vi "generate error.vi"() -> ()   [LabVIEW 2021, in "CIFCorePlugin.lvclass"]
uses:
  CIFCore/CIFCorePlugin/CIFCorePlugin.lvclass
  <vilib>/Utility/error.llb/DialogType.ctl
panel:
  out "call chain":string[](array[string])
  out "Callers' Names":string[](array[string])
  out "error out 2":errorcluster
  out "Name":string
  out "VI Name":string
  out "code out":i32 format="%0.0f"
  out "source out":string
  out "message":string=" INSTRUCTIONS:\r\rNormal Use:  When using subVIs that incorporate the error in/error out (or error I/O) structure, place this handler where you want to inform the user of an error, typically at the end of the I/O data path, as the last action of the program.  If the error in error? is ERROR, the handler creates a message describing the error and its source.  If the type of dialog = 1 (default), the message is displayed to the user, who can only acknowedge it.  If the type = 2, the user can acknowledge the message or abort execution; aborting a program with active I/O is not recommended.  If the type = 0, no message is displayed; this is used to process the error programmatically, and the error out cluster elements are wired to individual terminals for that reason.  \r\rOther Use:\n\r\nlocal testing.  To test the error code of a subVI or function that does not have the error I/O structure, you can wire its error code and a source string to the local error code and error source inputs.  If error in error? indicates no error and error code is not equal to 0, the local code and source are substituted for the error in values, and error? is set TRUE (ERROR)."
  out "error out":errorcluster
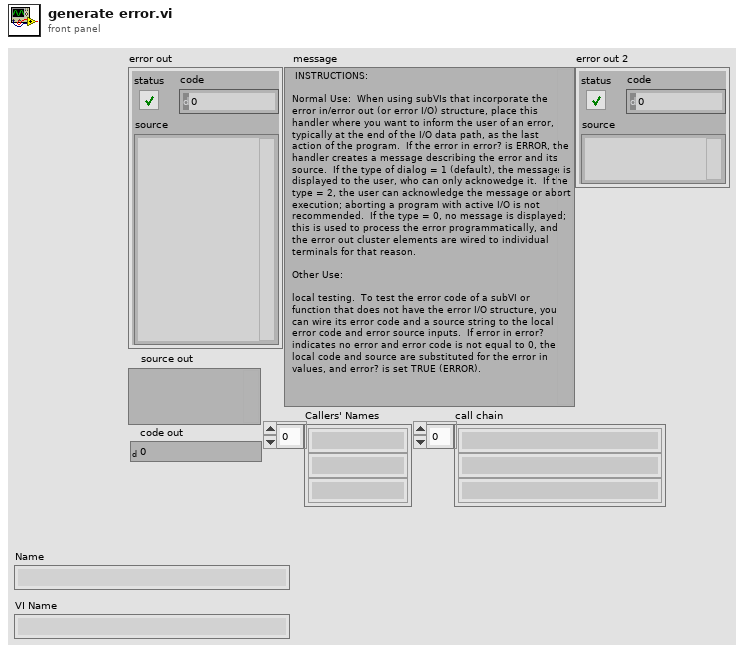
[diagram p1: front panel]
types:
  T1 = typedef "DialogType.ctl" = u16
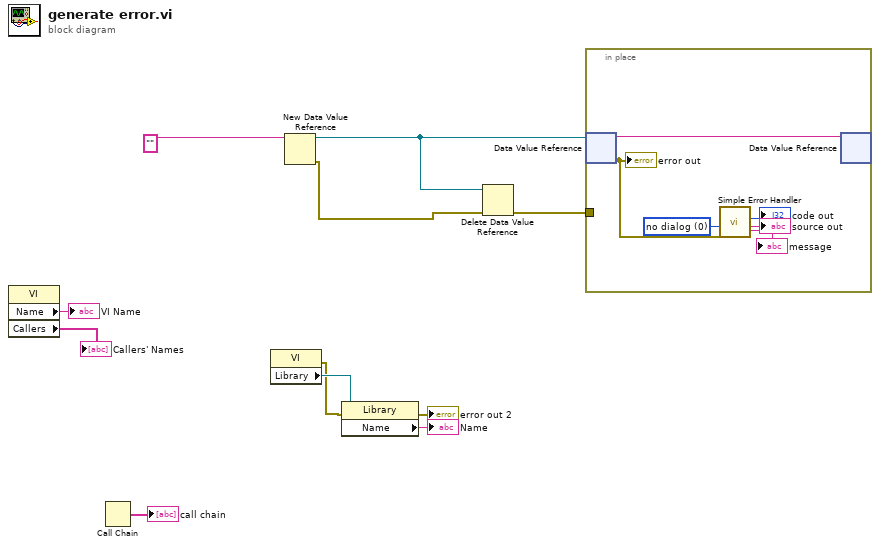
[diagram p0: block diagram]
diagram:
  n1 = property class="VI"() -> ("Name"=→"VI Name":string, "Callers"=→"Callers' Names":string[])  [unwired: 2 in, 2 out]
  n2 = Call Chain() -> (call chain=→"call chain":string[])
  n3 = property class="VI"() -> (error out=w4:errorcluster, "Library"=w6:refnum<vi>)  [unwired: 2 in, 1 out]
  n4 = New Data Value Reference(data value="") -> (data value reference=w9:refnum<data-value>, error out=w11:errorcluster)  [unwired: 1 in]
  n5 = property class="Library"(reference=w6, error in=w4) -> (error out=→"error out 2":errorcluster, "Name"=→"Name":string)  [unwired: 1 out]
  n6 = Delete Data Value Reference(data value reference=w9, error in=w11) -> (error out=w8:errorcluster)  [unwired: 1 out]
  n7 = in-place {
    in-place-border: w8 -> [_]
    w15 = T1 0 items=["no dialog", "OK message", "continue or stop message", "OK message + warnings", "continue/stop + warnings"] ("type of dialog (OK msg:1)")
    n8 = in-place-dvr #1(w9) -> (w17:string, w16:errorcluster)
    "error out" <- w16
    n9 = call <vilib>:"Simple Error Handler.vi"("type of dialog (OK msg:1)"=w15, "error in (no error)"=w16) -> ("code out"=→"code out":i32, "source out"=→"source out":string, "message"=→"message":string)  [unwired: 3 in, 2 out]
    n10 = in-place-dvr #1(w17) -> ()  [unwired: 2 out]
  }
